vi "Enable_Relays.vi"(8 "error in (no error)":errorcluster caption="entrée d'erreur (pas d'erreur)", 11 "Class Relay_Board 16_Relay_R4D3D16 en entrée":refnum<class "Class Relay_Board 8_Relay_N4D8B08.lvclass">) -> (0 "error out":errorcluster caption="sortie d'erreur", 3 "Class Relay_Board 16_Relay_R4D3D16 en sortie":refnum<class "Class Relay_Board 8_Relay_N4D8B08.lvclass">)   [LabVIEW 2020, in "Library Instrument & Equipement.lvlib" / "Library Relay_Board.lvlib" / "Class Relay_Board 8_Relay_N4D8B08.lvclass"]
uses:
  Class Relay_Board 8_Relay_N4D8B08.lvclass
  C:/Users/ngarcin/OneDrive - Altyor/Standard TB/Class/Relay_Board/Relay_Board (Default)/Class Relay_Board (Default).lvclass
  Class Relay_Board 8_Relay_N4D8B08.lvclass/Class Relay_Board 8_Relay_N4D8B08.ctl
  Commun VI/TypeDef/Liste Error.ctl
  Modbus/Modbus.lvclass
  Commun VI/Library Commun.lvlib
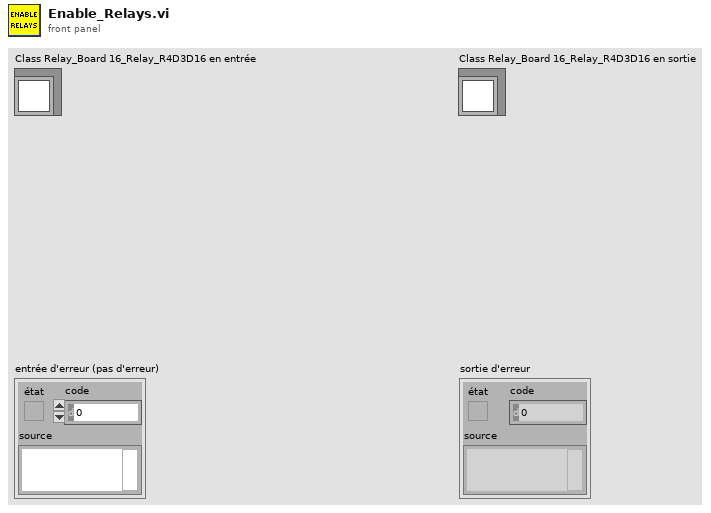
[diagram p1: front panel]
types:
  T1 = typedef "Library Commun.lvlib/Liste Error.ctl" = enum16{"Firebase Driver - Get Document", "Firebase Driver - Get Document With Where", "Firebase Driver - Delete Document", "Firebase Driver - Set Document", "Firebase Driver - Update Document", "Firebase Altyor - Search Document Bench", "Firebase Altyor - Class Not in Firebase", "Spectrum_Analyser - Timeout", "Relay Board - Qty Relay", "DIO - Pb Funtion", "Power_Supply - Peripherical not find", "Mutimeter - Peripherical not find", "Instrument - Function Not Used", "Instrument - Instrument name not specified", "Instrument - Allready Initialised", "Instrument - TimeOut", "Instrument - the instrument must be Initialise before", "Instrument - Frame Not received", "Instrument - Frame Nok", "Test - Initialise the File_for_Save", "Test - Timeout", "Test - Cmd Error", "FGV - Variable ", "BDD FireBase - Define Class", "SN - Class Not Define"}
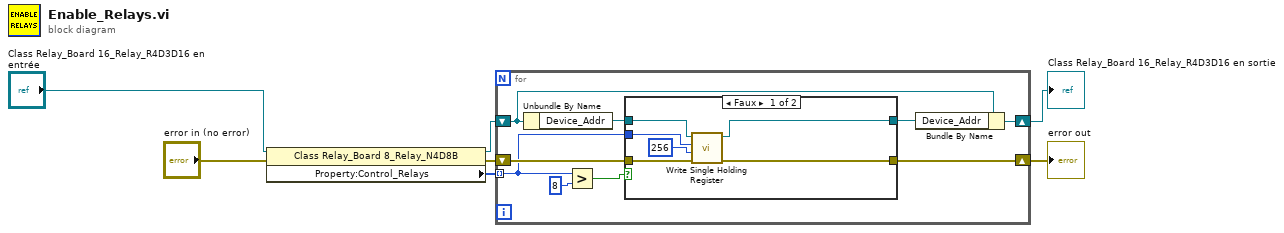
[diagram p0: block diagram]
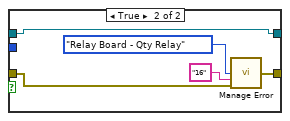
[diagram p2: hidden frame]
diagram:
  n1 = property class="Class Relay_Board 8_Relay_N4D8B"(reference="Class Relay_Board 16_Relay_R4D3D16 en entrée", error in="error in (no error)") -> (reference out=w5:refnum<class "Class Relay_Board 8_Relay_N4D8B08.lvclass">, error out=w1:errorcluster, "Property:Control_Relays"=w2:u8[])
  n2 = for {
    shift-right: [w15] -> w3
    shift-left: w1 -> [w16]
    tunnel: w2 -> [w13] mode=indexing
    shift-right: [w9] -> w4
    shift-left: w5 -> [w11]
    n3 = Unbundle By Name(w11) -> ("Device_Addr"=w8:refnum<class "Modbus.lvclass">)
    n4 = Greater?(x=w13, y=u8 8) -> (0:w12:bool)
    n5 = case shown="Faux" w12 {
      tunnel: w16 -> [w22 w23]
      tunnel: w13 -> [w21 _]
      tunnel: [w17 w25] -> w15
      tunnel: [w19 w24] -> w10
      tunnel: w8 -> [w18 w24]
      frame False {
        n6 = call "Write Single Holding Register.vi"("error in (no error)"=w22, "value"=u16 256, "address"=w21, "MODBUS in"=w18) -> ("error out"=w17:errorcluster, "MODBUS Out"=w19:refnum<class "Modbus.lvclass">)  [unwired: 6 in]
      }
      frame True {
        n7 = call "Manage Error.vi"("Code Erreur"=Liste_Error."Relay Board - Qty Relay", "Text"="16", "error in (no error)"=w23) -> ("error out"=w25:errorcluster)  [unwired: 12 in]
      }
    }
    n8 = Bundle By Name(cluster=w11, "Device_Addr"=w10) -> (w9:refnum<class "Class Relay_Board 8_Relay_N4D8B08.lvclass">)
  }
  "error out" <- w3
  "Class Relay_Board 16_Relay_R4D3D16 en sortie" <- w4
